vi "Brushless DC Motor.vi"(1 "Action":T4=enum."Identify", 2 "Parameters":variant) -> (6 "Output":variant, 7 "Stop":bool)   [LabVIEW 2019]
doc: "This VI reads a single reading from a Keithley 2001 multimeter. The stop boolean is always false. If no reading is obtained a single zero is returned.\nScott Hannahs, NHMFL-FSU, Nov 1993"
uses:
  Sub Controls/Scan Output.ctl
  Sub Controls/Instrument IDN.ctl
  Sub Controls/User Event Command.ctl
  Sub Controls/Instrument Actions.ctl
  Sub Controls/Instrument Match.ctl
  Sub Controls/Public.ctl
panel:
  in  "Rotator":T1(ring)
  in  "Index":i32
  in  "Wait After Setting":dbl=5.0 format="%<%M:%S>t"
  in  "Time":dbl=1200.0 format="%<%H:%M:%S>t"
  in  "End Value":dbl=20.0
  in  "Step Size":dbl=1.0
  in  "Mode":bool=TRUE
  out "Title":string
  in  "Public":T2
  in  "Address":u16(ring)
  out "Model":string
  in  "Instruments":T3[](array[typedef])=[{"Model"="DS360", "Manufacturer"="StanfordResearchSystems", "Term Character"="", "Wait Time (mS)"=0, "Wait for SRQ"=FALSE, "Type"="Func. Gen."}, {"Model"="SR830", "Manufacturer"="Stanford_Research_Systems", "Term Character"="", "Wait Time (mS)"=0, "Wait for SRQ"=FALSE, "Type"="Func. Gen."}]
  out "Measurement":dbl[](array[numeric]) format="%^_7e"
  in  "VISA resource name":refnum<visa-resource-name>
  # "Term Char"
  # "Wait Time (mS)"
  # "Wait for SRQ?"
  # "Type"
  # "Manufacturer"
  # "Model"
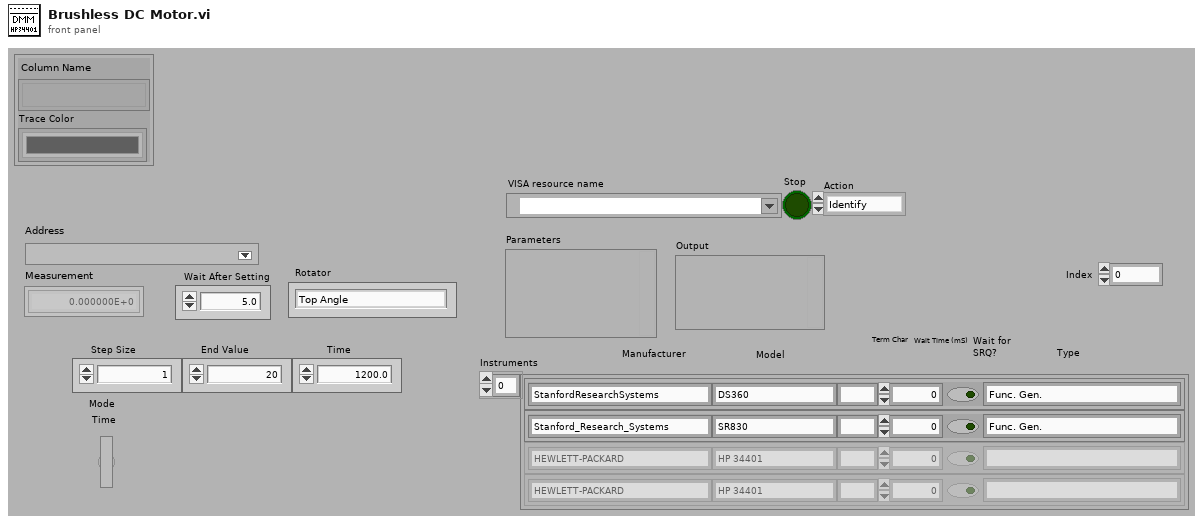
[diagram p1: front panel]
types:
  T1 = enum16{"Top Angle", "Dilution Fridge SCM 1", "System A SCM 2", "System B 50 mm Magnet", "He-3 32 mm Magnet", "Portable Dil Fridge Rotator", "Linear Position", "System E Probe 1"}
  T2 = typedef "Public.ctl" = cluster{"Column Name":string[], "Trace Color":u32[]}
  T3 = typedef "Instrument Match.ctl" = cluster{"Model":string, "Manufacturer":string, "Term Character":string, "Wait Time (mS)":u32, "Wait for SRQ":bool, "Type":string}
  T4 = typedef "Instrument Actions.ctl" = enum16{"Scan", "Identify", "New", "Configure", "Initialize", "Test", "Read", "Close"}
  T5 = typedef "Scan Output.ctl" = cluster{"Manufacturer":string, "Model":string, "Info":string, "Revision":string, "error out":errorcluster}
  T6 = typedef "Instrument IDN.ctl" = cluster{"VISA Address":string, "Status":u16, "Manufacturer":string, "Model":string, "Info":string, "Info 2":string, "Misc Data":variant}
  T7 = typedef "User Event Command.ctl" = enum32{"Stop Config"}
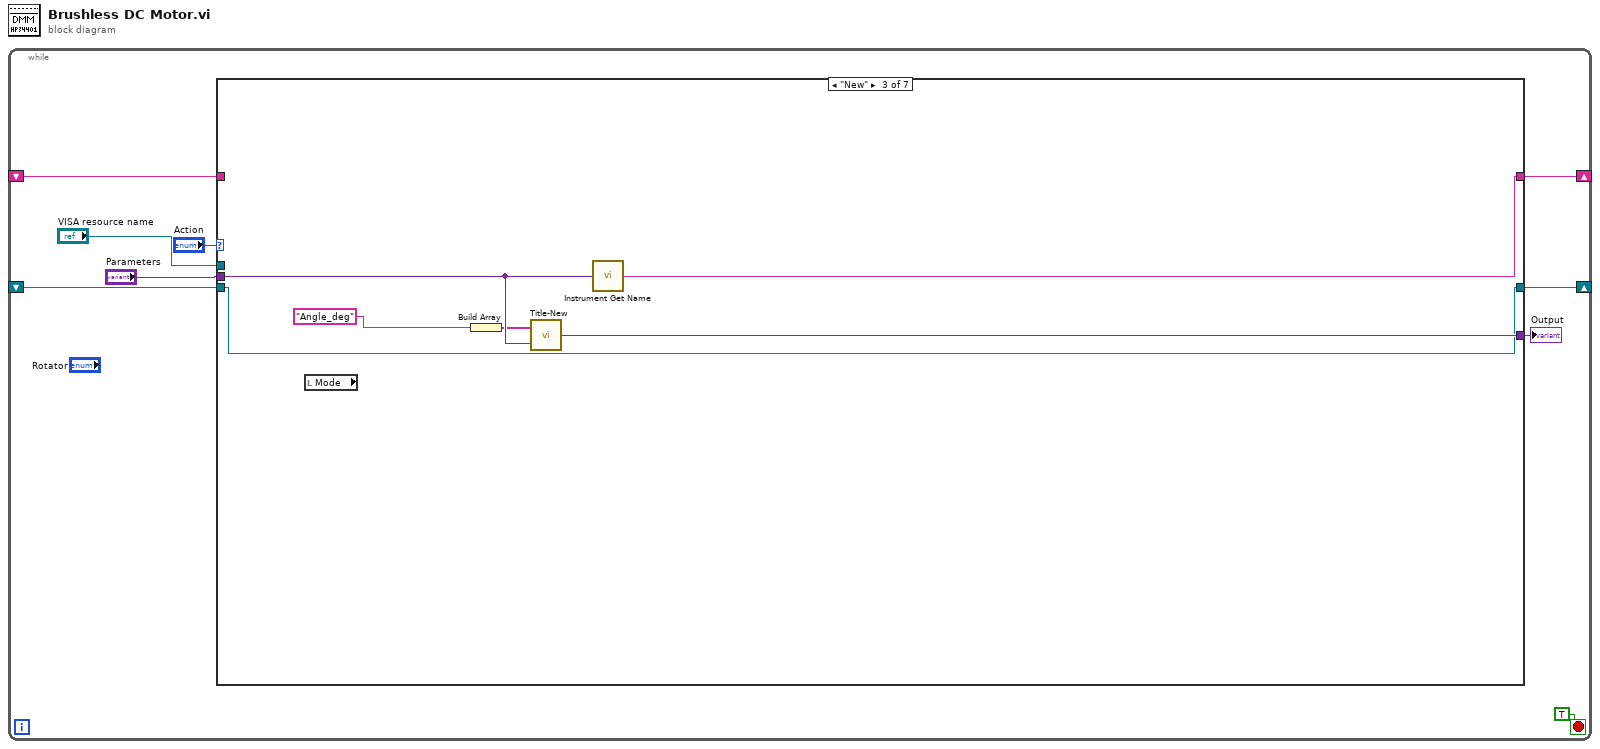
[diagram p0: block diagram]
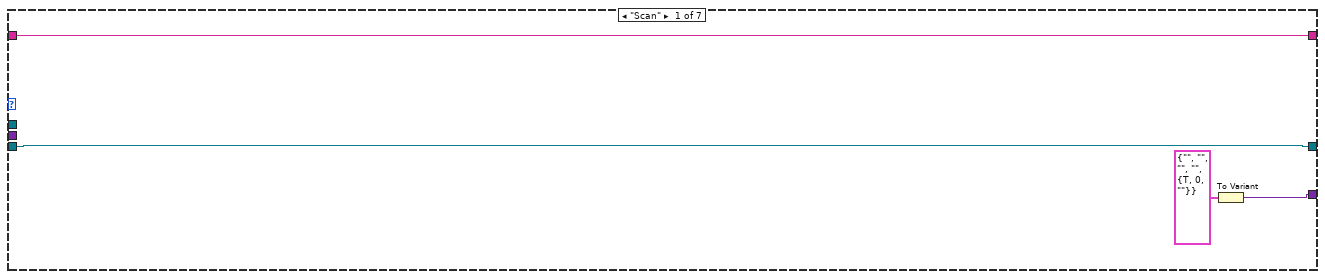
[diagram p2: hidden frame]
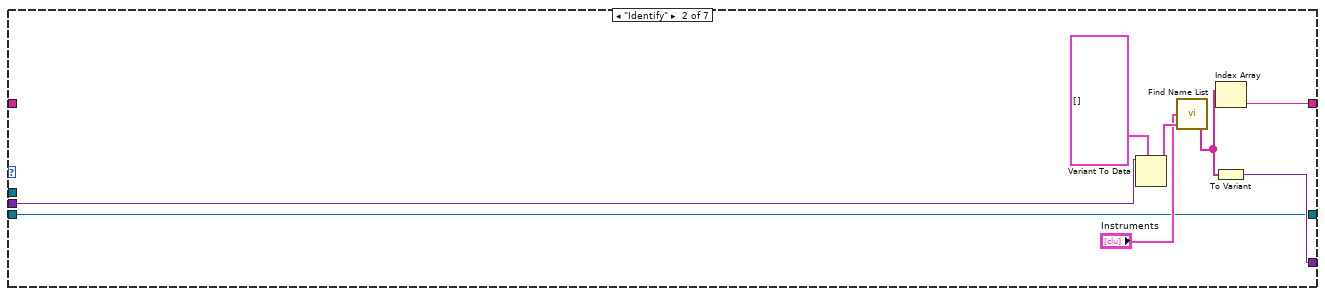
[diagram p3: hidden frame]
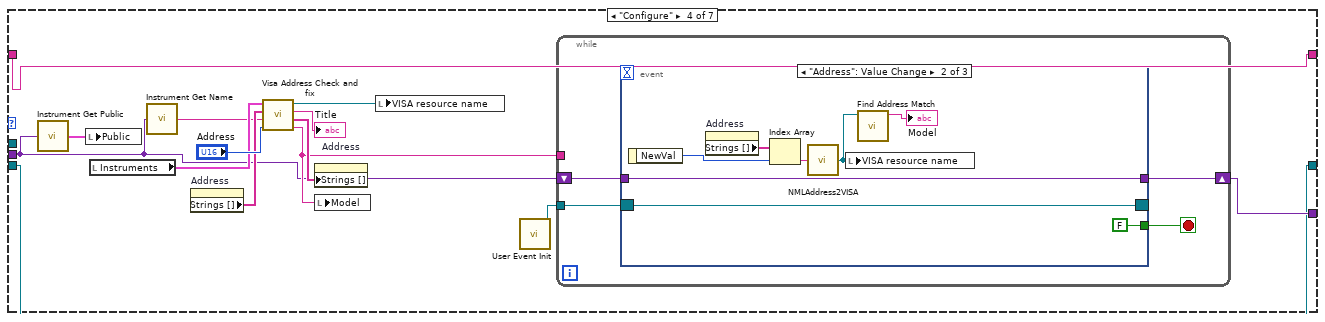
[diagram p4: hidden frame]
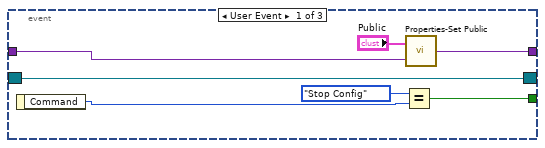
[diagram p5: hidden frame]
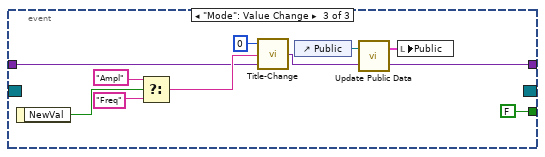
[diagram p6: hidden frame]
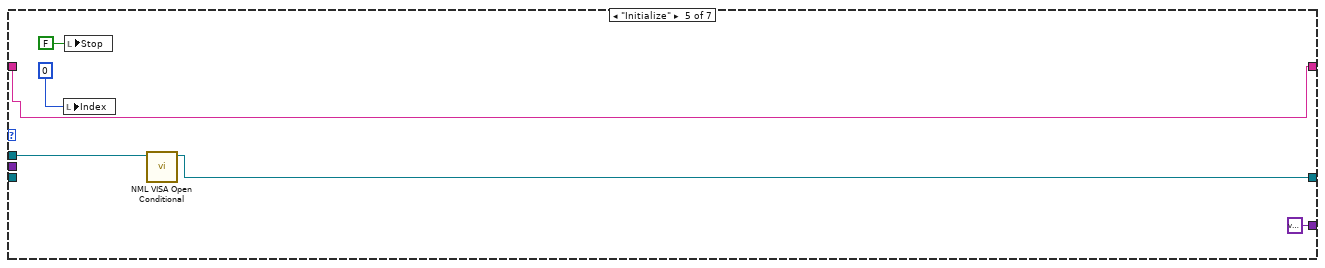
[diagram p7: hidden frame]
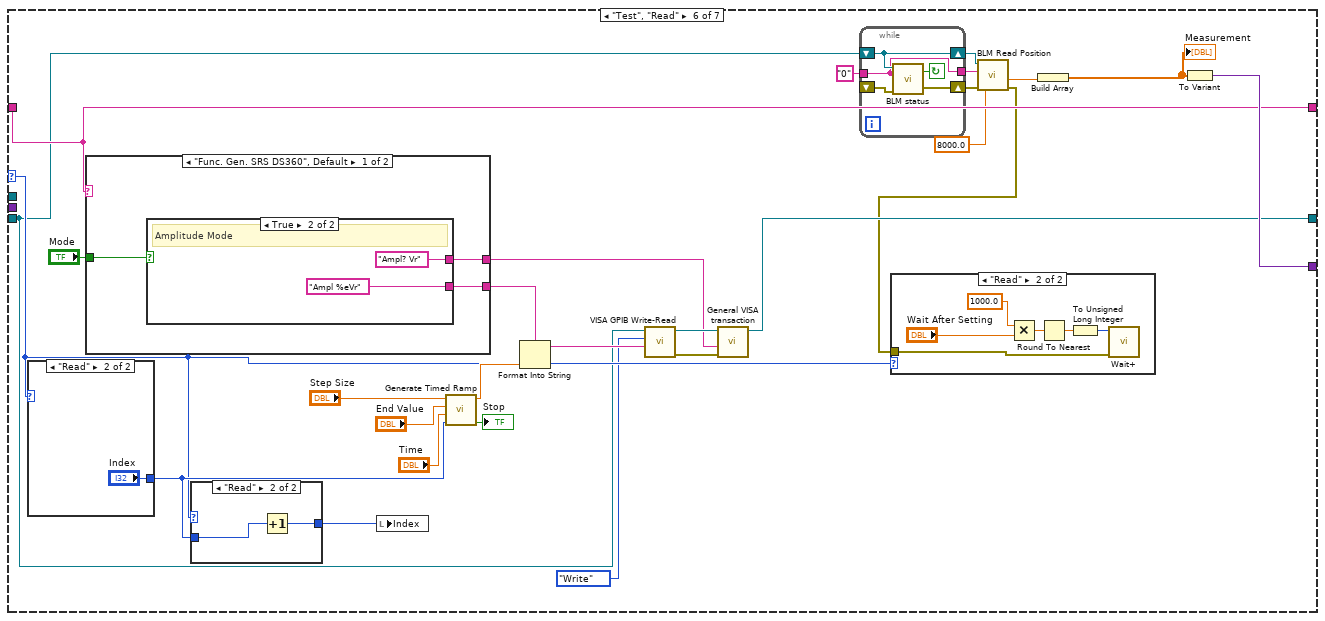
[diagram p8: hidden frame]
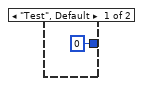
[diagram p11: hidden frame]
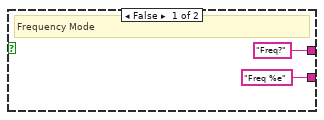
[diagram p12: hidden frame]
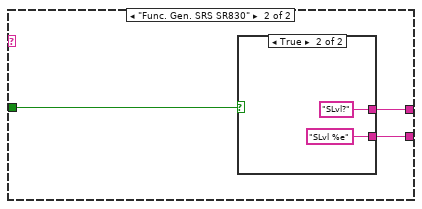
[diagram p13: hidden frame]
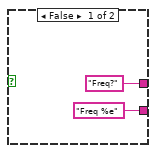
[diagram p14: hidden frame]
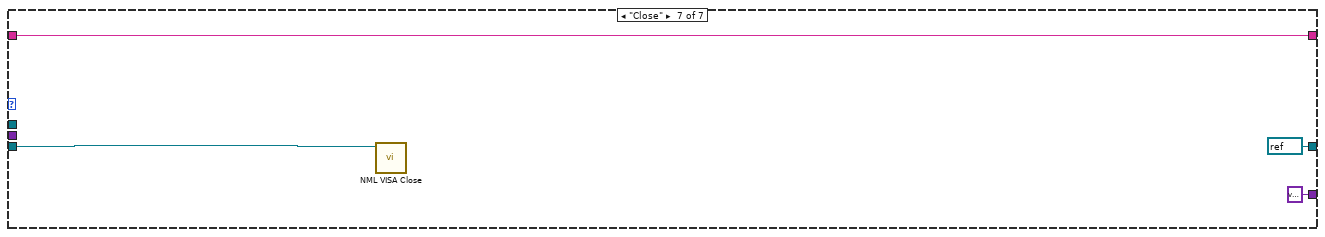
[diagram p15: hidden frame]
diagram:
  n1 = while {
    shift-right: [w5] -> _
    shift-left: _ -> [w4]
    shift-right: [w2] -> _
    shift-left: _ -> [w1]
    stop <- TRUE stop-if-true
    n2 = case shown="\"New\"" "Action" {
      selector: "Action" -> [_ _ _ _ _ w93 _]
      tunnel: [w13 w21 w27 w35 variant ("Variant") w104 variant ("Variant")] -> w7
      tunnel: "VISA resource name" -> [_ _ _ _ w77 _ _]
      tunnel: [w12 w16 w23 w28 w75 w92 w137] -> w5
      tunnel: w4 -> [w12 _ _ w28 w75 w92 w137]
      tunnel: "Parameters" -> [_ w20 w25 w31 _ _ _]
      tunnel: [w11 w14 w26 w32 w74 w103 refnum<visa-resource-name> refnum ("Open VISA Resource name")] -> w2
      tunnel: w1 -> [w11 w14 w26 w32 _ w85 w135]
      frame "Scan" {
        n3 = To Variant(anything=T5 {"Manufacturer"="", "Model"="", "Info"="", "Revision"="", "error out"={"status"=TRUE, "code"=0, "source"=""}} ("Scan Output")) -> (Variant=w13:variant)
      }
      frame "Identify" {
        n4 = Variant To Data(type=T6[] [], Variant=w20) -> (data=w18:T6[])  [unwired: 1 in, 1 out]
        n5 = call "Find Name List.vi"("Bus Scan"=w18, "Instruments"="Instruments") -> ("Names"=w15:string[])  [unwired: 1 in]
        n6 = Index Array(array=w15) -> (element=w16:string)  [unwired: 1 in]
        n7 = To Variant(anything=w15) -> (Variant=w21:variant)
      }
      frame "New" {
        n8 = local read "Mode"() -> ()  [unwired: 1 out]
        n9 = Build Array("Angle_deg") -> (w24:string[])
        n10 = call "Title-New.vi"("Parameters"=w25, "Array"=w24) -> ("Instrument Prop"=w27:variant)
        n11 = call "Instrument Get Name.vi"("Parameters"=w25) -> ("Type"=w23:string)
      }
      frame "Configure" {
        n12 = call "Instrument Get Public.vi"("Variant"=w31) -> ("Public"=w36:T2)
        n13 = local write "Public"(w36) -> ()
        n14 = local read "Instruments"() -> (w38:T3[])
        n15 = call "Instrument Get Name.vi"("Parameters"=w31) -> ("Type"=w30:string)
        n16 = property on="Address" class="Ring (strict)"() -> ("Strings []"=w39:string[])  [unwired: 2 in, 2 out]
        n17 = call "Visa Address Check and fix.vi"("Address"="Address", "Name"=w30, "NML Addresses"=w39, "Instruments"=w38) -> ("Model"=w37:string, "NML Addresses"=w41:string[], "Title"=→"Title":string, "VISA resource name"=w33:refnum<visa-resource-name>)  [unwired: 2 out]
        n18 = property on="Address" class="Ring (strict)"("Strings []"=w41) -> ()  [unwired: 2 in, 2 out]
        n19 = local write "Model"(w37) -> ()
        n20 = local write "VISA resource name"(w33) -> ()
        n21 = call "User Event Init.vi"() -> ("Event Registration Refnum"=w34:refnum<event-registration>)  [unwired: 14 in, 1 out]
        n22 = while {
          tunnel: w37 -> [_]
          tunnel: w34 -> [w42]
          shift-right: [w45] -> w35
          shift-left: w31 -> [w43]
          stop <- w44 stop-if-true
          n23 = event shown="[1] \"Address\": Value Change" {
            selector: w42 -> [w46 w54 _]
            dyn-events: [w46 w54 _] -> _
            timeout: _ -> [_ _ _]
            tunnel: [w50 w55 w63] -> w45
            tunnel: [w48 FALSE FALSE] -> w44
            tunnel: w43 -> [w51 w55 w66]
            event User Event {
              n24 = event-data() -> ("Command"=w52:T7)  [unwired: 1 in]
              n25 = Equal?(x=User_Event_Command."Stop Config", y=w52) -> (x = y?=w48:bool)
              n26 = call "Properties-Set Public.vi"("Variant"=w51, "New Public"="Public") -> ("Variant 2"=w50:variant)
            }
            event "Address": Value Change {
              n27 = event-data() -> ("NewVal"=w60:u16)  [unwired: 1 in]
              n28 = property on="Address" class="Ring (strict)"() -> ("Strings []"=w57:string[])  [unwired: 2 in, 2 out]
              n29 = Index Array(array=w57, index=w60) -> (element=w58:string)
              n30 = call "NMLAddress2VISA.vi"("NML Address"=w58) -> ("VISA resource name"=w53:refnum<visa-resource-name>)
              n31 = local write "VISA resource name"(w53) -> ()
              n32 = call "Find Address Match.vi"("VISA resource name"=w53) -> ("Model"=→"Model":string)  [unwired: 3 in, 3 out]
            }
            event "Mode": Value Change {
              n33 = event-data() -> ("NewVal"=w69:bool)  [unwired: 1 in]
              n34 = Select(t="Ampl", s=w69, f="Freq") -> (s? t:f=w68:string)
              n35 = call "Title-Change.vi"("Parameters"=w66, "New Title"=w68, "Index"=0) -> ("Variant"=w64:variant)
              n36 = control-ref of="Public"() -> (w61:refnum<vi>)
              n37 = call "Update Public Data.vi"("Variant In"=w64, "Public 2"=w61) -> ("Variant Out"=w63:variant, "Public"=w62:T2)
              n38 = local write "Public"(w62) -> ()
            }
          }
        }
      }
      frame "Initialize" {
        n39 = local write "Index"(0 ("Index")) -> ()
        n40 = local write "Stop"(FALSE ("Stop")) -> ()
        n41 = call "NML VISA Open Conditional.vi"("VISA resource name"=w77) -> ("dup VISA Session"=w74:refnum<visa-resource-name>)  [unwired: 8 in, 2 out]
      }
      frame "Test", "Read" {
        n42 = case shown="\"Read\"" w93 {
          tunnel: [0 ("Index") "Index"] -> w95
          frame "Test", Default {
          }
          frame "Read" {
          }
        }
        n43 = case shown="\"Func. Gen. SRS DS360\", Default" w92 {
          tunnel: [w122 w130] -> w89
          tunnel: "Mode" -> [w121 w129]
          tunnel: [w123 w128] -> w90
          frame "Func. Gen. SRS DS360", Default {
            n44 = case shown="True" w121 {
              tunnel: ["Freq %e" ("f") "Ampl %eVr"] -> w122
              tunnel: ["Freq?" ("f") "Ampl? Vr"] -> w123
              frame False {
                # "Frequency Mode"
              }
              frame True {
                # "Amplitude Mode"
              }
            }
          }
          frame "Func. Gen. SRS SR830" {
            n45 = case shown="True" w129 {
              tunnel: ["Freq %e" ("f") "SLvl %e"] -> w130
              tunnel: ["Freq?" ("f") "SLvl?"] -> w128
              frame False {
              }
              frame True {
              }
            }
          }
        }
        n46 = case shown="\"Read\"" w93 {
          tunnel: w95 -> [w116 w118]
          tunnel: [w116 w117] -> w94
          frame "Test", Default {
          }
          frame "Read" {
            n47 = Increment(x=w118) -> (x+1=w117:i32)
          }
        }
        n48 = local write "Index"(w94) -> ()
        n49 = call "Generate Timed Ramp.vi"("Point #"=w95, "Time (Hr:Min:Sec)"="Time", "Stop"="End Value", "Start"="Step Size") -> ("Stop"=→"Stop":bool, "Output"=w98:dbl)  [unwired: 1 in, 2 out]
        n50 = Format Into String(format string=w89, w98) -> (resulting string=w88:string)  [unwired: 2 in, 1 out]
        n51 = call "VISA GPIB Write-Read.vi"("Command"=w88, "Action"=enum16{"Write", "Read", "Write & Read"}."Write", "VISA resource name"=w85) -> ("error out"=w96:errorcluster, "dup VISA Session"=w97:refnum<visa-resource-name>)  [unwired: 5 in, 2 out]
        n52 = call "General VISA transaction.vi"("error in (no error)"=w96, "Command String"=w90, "VISA Session"=w97) -> ("dup VISA Session"=w103:refnum<visa-resource-name>)  [unwired: 3 in, 5 out]
        n53 = while {
          shift-right: [w108] -> w86
          shift-left: w85 -> [w108]
          shift-right: [w107] -> w84
          shift-left: _ -> [w106]
          tunnel: "0" ("Motor Address") -> [w105]
          tunnel: [w105] -> w82
          stop <- w109 continue-if-true
          n54 = call "BLM status.vi"("error in (no error)"=w106, "Motor Address"=w105, "Porty Address"=w108) -> ("error out"=w107:errorcluster, "Motor is moving"=w109:bool)  [unwired: 1 in]
        }
        n55 = call "BLM Read Position.vi"("error in (no error)"=w84, "Steps/rot"=8000.0, "Motor Address"=w82, "Port Address"=w86) -> ("error out"=w78:errorcluster, "Response"=w80:dbl)  [unwired: 2 out]
        n56 = case shown="\"Read\"" w93 {
          tunnel: w78 -> [_ w115]
          frame "Test", Default {
          }
          frame "Read" {
            n57 = Multiply(x=1000.0, y="Wait After Setting") -> (x*y=w113:dbl)
            n58 = Round To Nearest(number=w113) -> (nearest integer value=w114:dbl)
            n59 = To Unsigned Long Integer(number=w114) -> (unsigned 32bit integer=w110:u32)
            n60 = call "Wait+.vi"("Error In"=w115, "milliseconds to wait"=w110) -> ()  [unwired: 4 in, 2 out]
          }
        }
        n61 = Build Array(w80) -> (w79:dbl[])
        "Measurement" <- w79
        n62 = To Variant(anything=w79) -> (Variant=w104:variant)
      }
      frame "Close" {
        n63 = call "NML VISA Close.vi"("VISA resource name"=w135) -> ()  [unwired: 10 in, 1 out]
      }
    }
    "Output" <- w7
  }
